vi "FRC Color Processing Low Goal Example.vi"() -> ()   [LabVIEW 2016]
uses:
  <vilib>/Rock Robotics/WPI/Camera/WPI_CameraSettings Read MJPG.ctl
  <vilib>/Rock Robotics/WPI/Camera/WPI_CameraImageSize.ctl
  <vilib>/vision/NI_Vision_Development_Module.lvlib
panel:
  out "Top Score":dbl
  out "Instructions:":string="Use Source to load image files from a directory, or use a USB or IP camera connected to your laptop.\nLED Color can encoded as HSL or related color modes. Calibrate to the same color as the strips being reflected to the camera.\nClick and draw a line in Original Image to auto-calibrate to the LED Color. You may need to widen Sat and Val.\nAnnotate controls whether to draw a rectangle around the markings.\n\nAdjust Score Cutoff to make the code more or less picky. Because the color is not very unique, you may need to increase the number of particles to keep from the mask. The diagram uses a Size Limit to ignore colored things that are too small. You may need to adjust it if you are targetting from far away.\n\nResults give you the distance to the target, the center and box in a normalized (-1 to 1) and pixel coordinates.\n\nBe sure to read about setting up camera exposure and brightness to help simplify your image and acquire color saturated images."
  in  "Color Mode":u16(ring)=3 items=["RGB", "HSL", "HSV", "HSI"]
  in  "Particles":dbl=10.0
  in  "Score Cutoff":dbl=50.0
  in  "Std Devs for Calibration":cluster{"H":dbl, "S":dbl, "V":dbl}={"H"=4.0, "S"=6.0, "V"=6.0}
  in  "image files":string[](array[string])
  out "Results":T1 {"Error" format="%#_3g"; "Pixels"."Rectangle"."Numeric 5" format="%#_3g"; "Pixels"."Rectangle"."Numeric 3" format="%#_3g"; "Pixels"."Rectangle"."Numeric 2" format="%#_3g"; "Pixels"."Rectangle"."Numeric" format="%#_3g"; "Normalized"."Rectangle"."Numeric 5" format="%#_2g"; "Normalized"."Rectangle"."Numeric 3" format="%#_2g"; "Normalized"."Rectangle"."Numeric 2" format="%#_2g"; "Normalized"."Rectangle"."Numeric" format="%#_2g"; "Normalized"."Center"."?" format="%#_3g"; "Normalized"."Center"."?" format="%#_3g"; "Distance (ft)" format="%#_3g"}
  in  "Source":enum32{"Files", "Camera"}(tab)
  in  "Images":i32(listbox)
  in  "Folder Location":path=path "C:/Program Files (x86)/National Instruments/LabVIEW 2016/examples/FRC/roboRIO/Vision/2017 Vision Example/Sample Images/Low Images"
  in  "Camera Settings":T2={"fps"=20, "compression"=30, "Image Size"=enum."320x240", "Config Shown"=FALSE}
  in  "Camera Address":string="USB 1"
  in  "Annotate":bool=TRUE
  out "Qualified Particles":i32
  in  "LED Color":T4={"Hue"={110.52399131877658, 148.6727294921875}, "Sat"={34.78571428571429, 255.0}, "Val"={91.07142857142858, 255.0}} {"Hue" scale=0.0..255.0 scale format="%#_3g"}
  out "Mask":T5(plugin-control)
  out "Original Image":T5(plugin-control)
  # "Legend:\n    Rectangle\n       Green - Good target, distance in ft\n       Red - Bad target\n    Orange Text - Score in %"
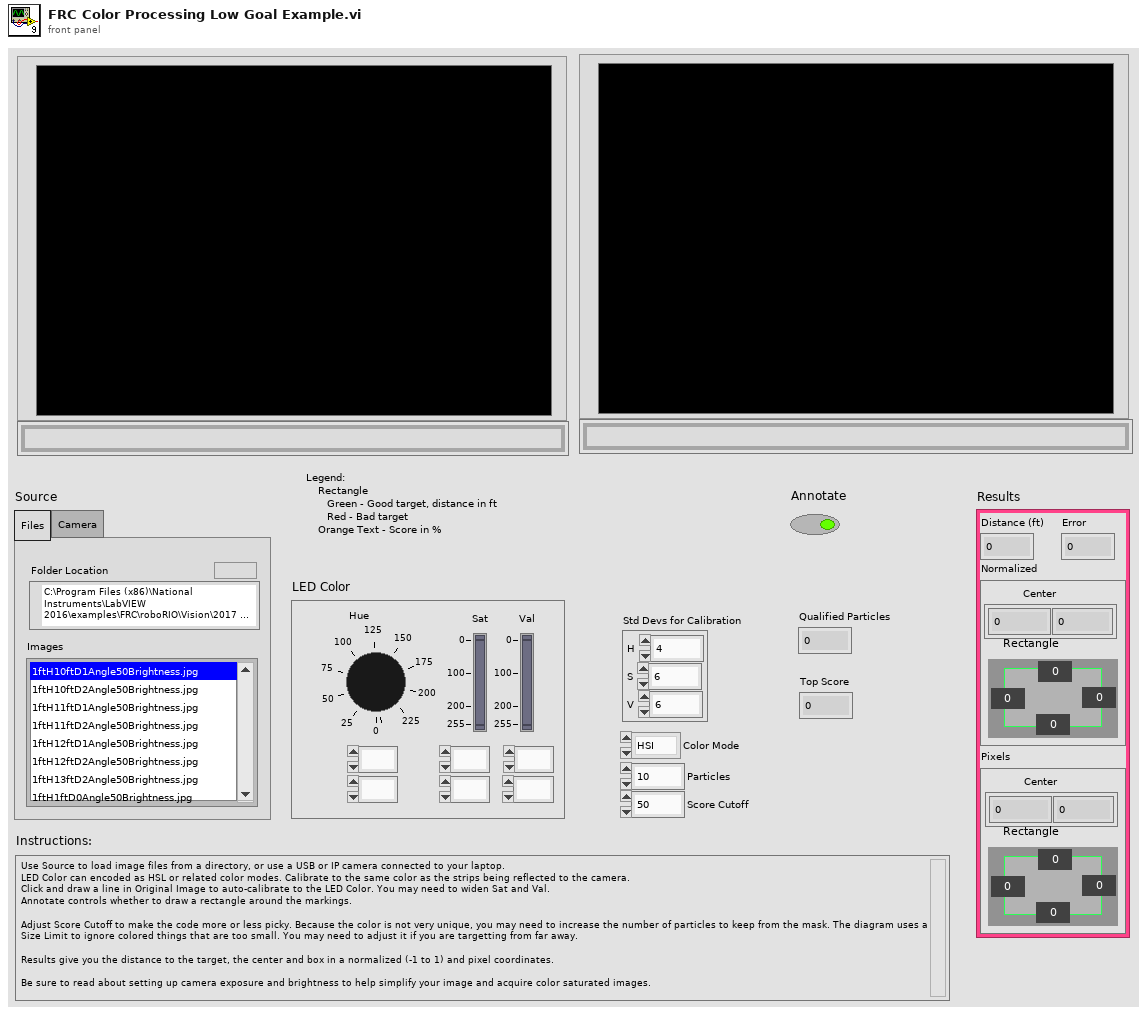
[diagram p1: front panel]
types:
  T1 = cluster{"Distance (ft)":dbl, "Error":dbl, "Normalized":cluster{"Center":cluster{dbl, dbl}, "Rectangle":cluster{"Numeric":dbl, "Numeric 2":dbl, "Numeric 3":dbl, "Numeric 5":dbl}}, "Pixels":cluster{"Center":cluster{dbl, dbl}, "Rectangle":cluster{"Numeric":dbl, "Numeric 2":dbl, "Numeric 3":dbl, "Numeric 5":dbl}}}
  T2 = typedef "WPI_CameraSettings Read MJPG.ctl" = cluster{"fps":i32, "compression":i32, "Image Size":T3, "Config Shown":bool}
  T3 = typedef "WPI_CameraImageSize.ctl" = enum16{"640x480", "320x240", "160x120", "Custom"}
  T4 = cluster{"Hue":cluster{dbl, dbl}, "Sat":cluster{dbl, dbl}, "Val":cluster{dbl, dbl}}
  T5 = typedef "IMAQ Image.ctl" = refnum<image>
  T6 = typedef "Particle Parameters" = i32
  T7 = typedef "Image Type" = u32
  T8 = cluster{cluster{dbl, dbl}, cluster{dbl, dbl}, cluster{dbl, dbl}}
  T9 = cluster{"Left":dbl, "Top":dbl, "Right":dbl, "Bottom":dbl}
  T10 = cluster{"Distance (ft)":dbl, "Score":dbl, "Normalized":cluster{"Center":cluster{dbl, dbl}, "Rectangle":cluster{"Numeric":dbl, "Numeric 2":dbl, "Numeric 3":dbl, "Numeric 5":dbl}}, "Pixels":cluster{"Center":cluster{dbl, dbl}, "Rectangle":cluster{"Numeric":dbl, "Numeric 2":dbl, "Numeric 3":dbl, "Numeric 5":dbl}}}
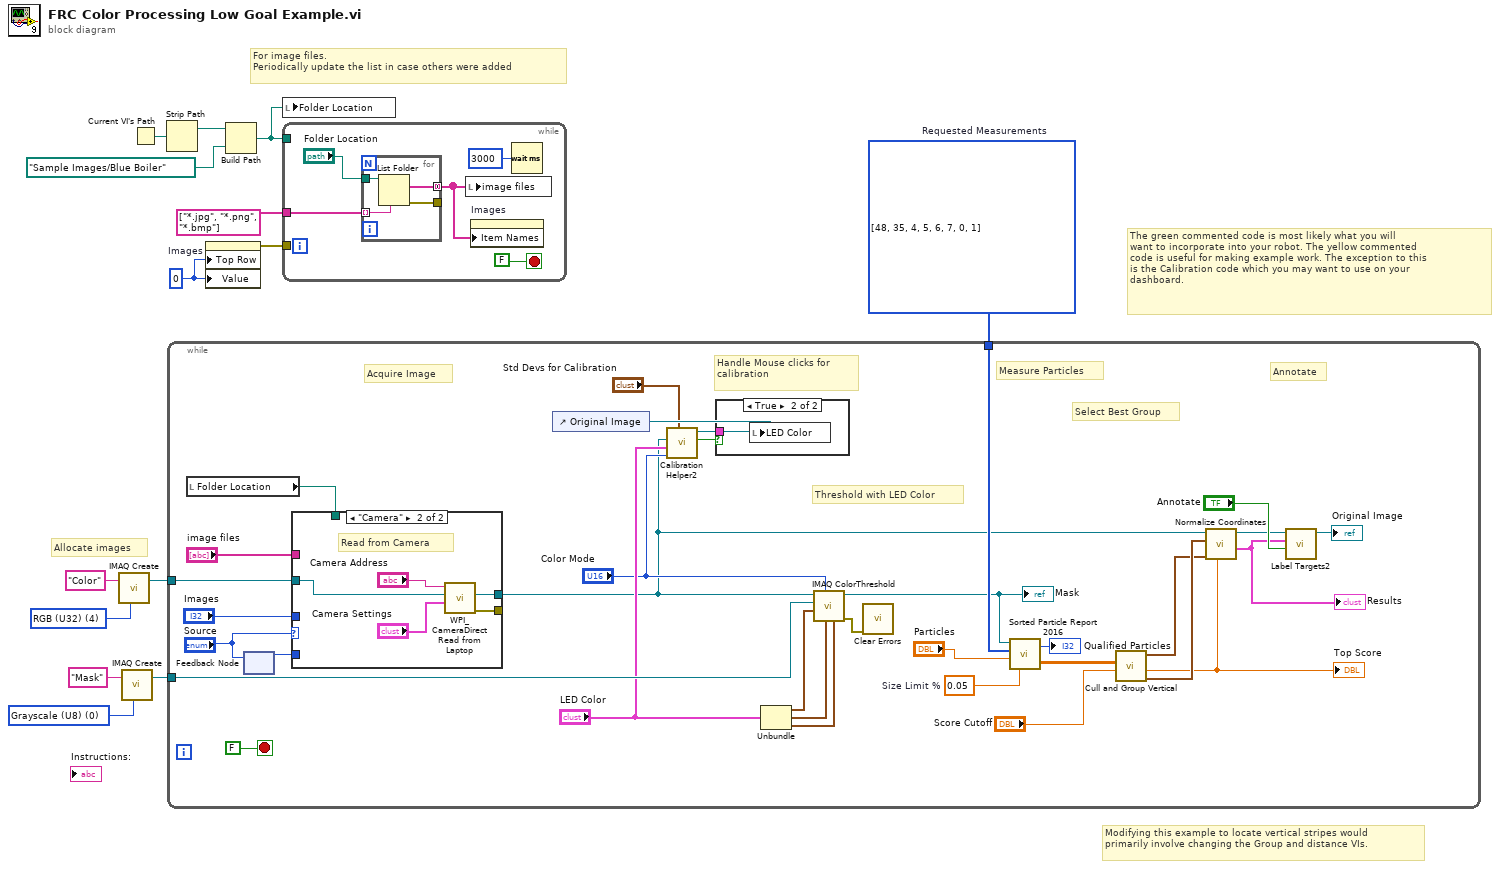
[diagram p0: block diagram]
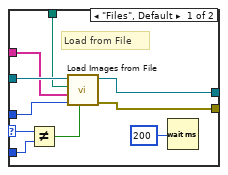
[diagram p3: hidden frame]
diagram:
  w2 = u32 0 ("milliseconds to wait")
  w8 = T6[] [48, 35, 4, 5, 6, 7, 0, 1] items=["Center of Mass X", "Center of Mass Y", "First Pixel X", "First Pixel Y", "Bounding Rect Left", "Bounding Rect Top", "Bounding Rect Right", "Bounding Rect Bottom", "Max Feret Diameter Start X", "Max Feret Diameter Start Y", "Max Feret Diameter End X", "Max Feret Diameter End Y", "Max Horiz. Segment Length Left", "Max Horiz. Segment Length Right", "Max Horiz. Segment Length Row", "-", "Bounding Rect Width", "Bounding Rect Height", "Bounding Rect Diagonal", "Perimeter", "Convex Hull Perimeter", "Holes' Perimeter", "Max Feret Diameter", "Equivalent Ellipse Major Axis", "Equivalent Ellipse Minor Axis", "Equivalent Ellipse Minor Axis (Feret)", "Equivalent Rect Long Side", "Equivalent Rect Short Side", "Equivalent Rect Diagonal", "Equivalent Rect Short Side (Feret)", "Average Horiz. Segment Length", "Average Vert. Segment Length", "Hydraulic Radius", "Waddel Disk Diameter", "-", "Area", "Holes' Area", "Particle & Holes' Area", "Convex Hull Area", "Image Area", "-", "Number of Holes", "Number of Horiz. Segments", "Number of Vert. Segments", "-", "Orientation", "Max Feret Diameter Orientation", "-", "% Area/Image Area", "% Area/(Particle & Holes' Area)", "Ratio of Equivalent Ellipse Axes", "Ratio of Equivalent Rect Sides", "-", "Elongation Factor", "Compactness Factor", "Heywood Circularity Factor", "Type Factor", "-", "Sum X", "Sum Y", "Sum XX", "Sum XY", "Sum YY", "Sum XXX", "Sum XXY", "Sum XYY", "Sum YYY", "-", "Moment of Inertia XX", "Moment of Inertia XY", "Moment of Inertia YY", "Moment of Inertia XXX", "Moment of Inertia XXY", "Moment of Inertia XYY", "Moment of Inertia YYY", "Norm. Moment of Inertia XX", "Norm. Moment of Inertia XY", "Norm. Moment of Inertia YY", "Norm. Moment of Inertia XXX", "Norm. Moment of Inertia XXY", "Norm. Moment of Inertia XYY", "Norm. Moment of Inertia YYY", "Hu Moment 1", "Hu Moment 2", "Hu Moment 3", "Hu Moment 4", "Hu Moment 5", "Hu Moment 6", "Hu Moment 7"]  # Requested Measurements
  w11 = T7 0 items=["Grayscale (U8)", "Grayscale (I16)", "Grayscale (SGL)", "Complex (CSG)", "RGB (U32)", "HSL (U32)", "RGB (U64)", "Grayscale (U16)"] ("Image Type")
  w13 = T7 4 items=["Grayscale (U8)", "Grayscale (I16)", "Grayscale (SGL)", "Complex (CSG)", "RGB (U32)", "HSL (U32)", "RGB (U64)", "Grayscale (U16)"] ("Image Type")
  # "Modifying this example to locate vertical stripes would\nprimarily involve changing the Group and distance VIs."
  # "The green commented code is most likely what you will\nwant to incorporate into your robot. The yellow commented\ncode is useful for making example work. The exception to this\nis the Calibration code which you may want to use on your\ndashboard."
  # "For image files.\nPeriodically update the list in case others were added"
  # "Allocate images"
  n1 = call "IMAQ Create"("Image Name"="Color", "Image Type"=w13) -> ("New Image"=w12:T5)  [unwired: 2 in, 2 out]
  n2 = call "IMAQ Create"("Image Name"="Mask", "Image Type"=w11) -> ("New Image"=w9:T5)  [unwired: 2 in, 2 out]
  n3 = Current VI's Path() -> (path=w7:path)
  n4 = Strip Path(path=w7) -> (stripped path=w5:path)  [unwired: 1 out]
  n5 = while {
    tunnel: w12 -> [w46]
    tunnel: w9 -> [w44]
    tunnel: w8 -> [w40]
    stop <- FALSE stop-if-true
    w38 = 0.05  # Size Limit %
    # "Handle Mouse clicks for\ncalibration"
    # "Measure Particles"
    # "Annotate"
    # "Select Best Group"
    # "Threshold with LED Color"
    # "Acquire Image"
    n6 = local read "Folder Location"() -> (w28:path)
    n7 = feedback-in #1("Source") -> ()
    n8 = feedback #1() -> (w26:enum32{"Files", "Camera"})  [unwired: 1 in]
    n9 = case shown="\"Camera\"" "Source" {
      selector: "Source" -> [w51 _]
      tunnel: [w57 w63] -> _
      tunnel: [w58 w62] -> w16
      tunnel: w46 -> [w56 w61]
      tunnel: "image files" -> [w53 _]
      tunnel: "Images" -> [w55 _]
      tunnel: w28 -> [w54 _]
      tunnel: w26 -> [w50 _]
      frame "Files", Default {
        # "Load from File"
        n10 = Not Equal?(x=w51, y=w50) -> (x != y?=w49:bool)
        n11 = call "Load Images from File.vi"("Force Load"=w49, "Images"=w55, "image files"=w53, "Folder Location"=w54, "Refnum in"=w56) -> ("error out"=w57:errorcluster, "Refnum out"=w58:T5)  [unwired: 5 in]
        n12 = Wait (ms)(milliseconds to wait=u32 200 ("delay (ms)")) -> ()  [unwired: 1 out]
      }
      frame "Camera" {
        # "Read from Camera"
        n13 = call <vilib>:"WPI_CameraDirect Read from Laptop.vi"("Camera Settings"="Camera Settings", "Image"=w61, "address"="Camera Address") -> ("error out"=w63:errorcluster, "Image Out"=w62:T5)  [unwired: 7 in]
      }
    }
    n14 = control-ref of="Original Image"() -> (w33:refnum<vi>)
    n15 = call "Calibration Helper2.vi"("Std Devs"="Std Devs for Calibration", "Color Mode"="Color Mode", "Color Components"="LED Color", "Image"=w16, "Image Ctl Refnum"=w33) -> ("Changed"=w32:bool, "output color"=w31:T8)  [unwired: 5 in]
    n16 = case shown="True" w32 {
      tunnel: w31 -> [_ w48]
      frame False {
      }
      frame True {
        n17 = local write "LED Color"(w48) -> ()
      }
    }
    n18 = Unbundle("LED Color") -> ("Hue"=w43:cluster{dbl, dbl}, "Sat"=w42:cluster{dbl, dbl}, "Val"=w41:cluster{dbl, dbl})
    n19 = call "IMAQ ColorThreshold"("Blue or Luma or Val or Inten Range"=w41, "Green or Sat Range"=w42, "Color Mode"="Color Mode", "Red or Hue Range"=w43, "Image Dst"=w44, "Image Src"=w16) -> ("error out"=w34:errorcluster, "Image Dst Out"=w23:T5)  [unwired: 4 in]
    "Mask" <- w23
    n20 = call <vilib>:"Clear Errors.vi"("error in (no error)"=w34) -> ()  [unwired: 5 in, 2 out]
    n21 = call "Sorted Particle Report 2016.vi"("Min Area Size %"=w38, "Particle Count Limit"="Particles", "Pixel Measurements"=w40, "Image in"=w23) -> ("Sorted Data"=w25:dbl[][], "Particles"=→"Qualified Particles":i32)
    n22 = call "Cull and Group Vertical.vi"("Score Cutoff"="Score Cutoff", "Sorted Data"=w25) -> ("Rect"=w22:T9, "Top Score"=w15:dbl, "Center"=w20:cluster{"X":dbl, "Y":dbl})  [unwired: 7 in]
    "Top Score" <- w15
    n23 = call "Normalize Coordinates.vi"("Score"=w15, "Center"=w20, "Bounding box"=w22, "Image in"=w16) -> ("Results"=w19:T10, "Image out"=w21:T5)  [unwired: 6 in]
    "Results" <- w19
    n24 = call "Label Targets2.vi"("Annotate"="Annotate", "Results"=w19, "Image in"=w21) -> ("Image out"=→"Original Image":T5)  [unwired: 8 in]
  }
  n25 = property on="Images" class="LstBox (strict)"("Top Row"=w2, "Value"=w2) -> (error out=w3:errorcluster)  [unwired: 2 in, 1 out]
  n26 = Build Path(base path=w5, name or relative path=path "Sample Images/Blue Boiler" ("Folder Location")) -> (appended path=w4:path)
  n27 = local write "Folder Location"(w4) -> ()
  n28 = while {
    tunnel: w4 -> [_]
    tunnel: w3 -> [_]
    tunnel: string[] ["*.jpg", "*.png", "*.bmp"] -> [w64]
    stop <- FALSE stop-if-true
    n29 = for {
      tunnel: [w72] -> w66 mode=concatenating
      tunnel: "Folder Location" -> [w71]
      tunnel: [w70] -> _
      tunnel: w64 -> [w69] mode=indexing
      n30 = List Folder(path=w71, pattern=w69) -> (filenames=w72:string[], error out=w70:errorcluster)  [unwired: 2 in, 2 out]
    }
    n31 = local write "image files"(w66) -> ()
    n32 = property on="Images" class="LstBox (strict)"("Item Names"=w66) -> ()  [unwired: 2 in, 2 out]
    n33 = Wait (ms)(milliseconds to wait=u32 3000) -> ()  [unwired: 1 out]
  }
